vi "ffc.vi"() -> ()   [LabVIEW 2025]
panel:
  out "sum":sgl
  out "x-y":dbl
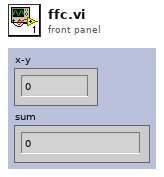
[diagram p1: front panel]
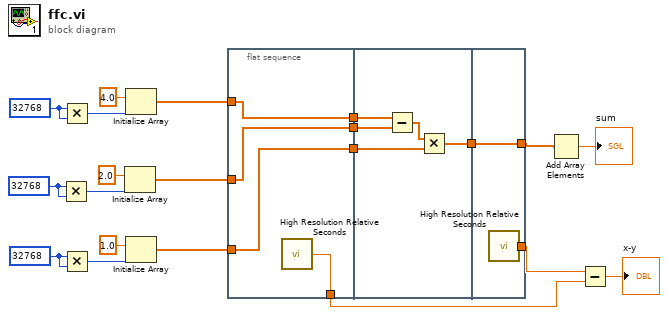
[diagram p0: block diagram]
diagram:
  w15 = 32768 ("x")
  w18 = 32768 ("x")
  w21 = 32768 ("x")
  n1 = Multiply(x=w18, y=w18) -> (x*y=w17:i32)
  n2 = Multiply(x=w21, y=w21) -> (x*y=w20:i32)
  n3 = Multiply(x=w15, y=w15) -> (x*y=w14:i32)
  n4 = Initialize Array(sgl 2.0 ("element"), w17) -> (w11:sgl[])
  n5 = Initialize Array(sgl 4.0 ("element"), w20) -> (w12:sgl[])
  n6 = Initialize Array(sgl 1.0 ("element"), w14) -> (w10:sgl[])
  n7 = flat-sequence {
    tunnel: w12 -> [w25]
    tunnel: w11 -> [w24]
    tunnel: w10 -> [w23]
    tunnel: [w25] -> w9
    tunnel: [w24] -> w8
    tunnel: [w23] -> w7
    tunnel: [w22] -> w4
    tunnel: w9 -> [w30]
    tunnel: w8 -> [w29]
    tunnel: w7 -> [w27]
    tunnel: [w26] -> w6
    tunnel: [w32] -> w2
    tunnel: w6 -> [w32]
    tunnel: [w31] -> w5
    frame #0 {
      n8 = call <vilib>:"High Resolution Relative Seconds.vi"() -> ("relative seconds"=w22:dbl)
    }
    frame #1 {
      n9 = Subtract(x=w30, y=w29) -> (x-y=w28:sgl[])
      n10 = Multiply(x=w28, y=w27) -> (x*y=w26:sgl[])
    }
    frame #2 {
      n11 = call <vilib>:"High Resolution Relative Seconds.vi"() -> ("relative seconds"=w31:dbl)
    }
  }
  n12 = Add Array Elements(numeric array=w2) -> (sum=→"sum":sgl)
  n13 = Subtract(x=w5, y=w4) -> (x-y=→"x-y":dbl)
